vi "Get Objects.vi"(8 "error in (no error)":errorcluster, 11 "Analyze Compound Results Base in":refnum<class "Analyze Compound Results Base.lvclass">) -> (0 "error out":errorcluster, 2 "Result Objs":refnum<class "Analyze Results Base.lvclass">[](array[class]), 3 "Analyze Compound Results Base out":refnum<class "Analyze Compound Results Base.lvclass">)   [LabVIEW 2014, in "Analyze Compound Results Base.lvclass"]
uses:
  Analyze Compound Results Base.lvclass
  Results Base/Analyze Results Base.lvclass
  Analyze Compound Results Base.lvclass/Analyze Compound Results Base.ctl
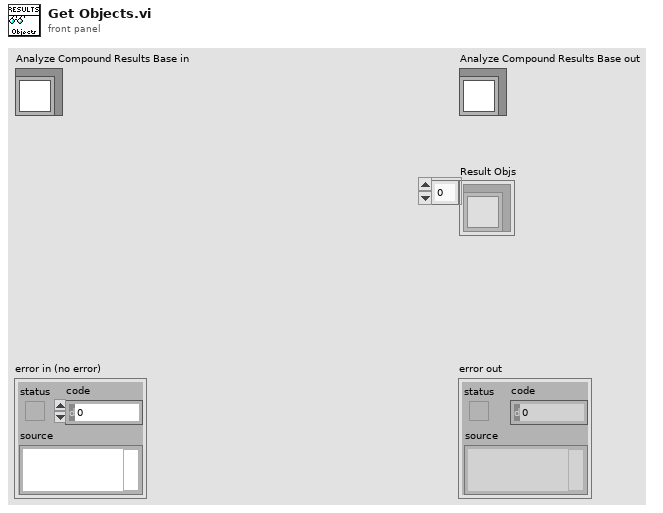
[diagram p1: front panel]
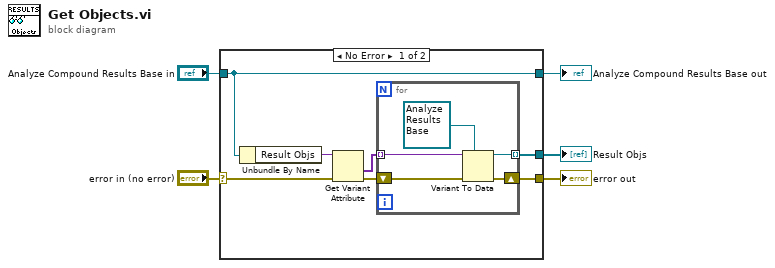
[diagram p0: block diagram]
diagram:
  n1 = case shown="No Error" "error in (no error)" {
    selector: "error in (no error)" -> [w8 w19]
    tunnel: [w7 w19] -> w4
    tunnel: [w12 w18] -> w2
    tunnel: "Analyze Compound Results Base in" -> [w12 w18]
    tunnel: [w6 _] -> w1
    frame No Error {
      n2 = Unbundle By Name(w12) -> ("Result Objs"=w11:variant)
      n3 = Get Variant Attribute(Variant=w11, error in=w8) -> (values=w10:variant[], error out=w9:errorcluster)  [unwired: 2 in, 2 out]
      n4 = for {
        tunnel: w10 -> [w17] mode=indexing
        shift-right: [w15] -> w7
        shift-left: w9 -> [w16]
        tunnel: [w13] -> w6 mode=indexing
        n5 = Variant To Data(error in=w16, type=refnum<class "Analyze Results Base.lvclass"> refnum ("Analyze Results Base.lvclass"), Variant=w17) -> (data=w13:refnum<class "Analyze Results Base.lvclass">, error out=w15:errorcluster)
      }
    }
    frame Error {
    }
  }
  "error out" <- w4
  "Analyze Compound Results Base out" <- w2
  "Result Objs" <- w1
